vi "Producer Comsumer pattern.vi"() -> ()   [LabVIEW 2024]
panel:
  in  "stop":bool
  in  "Enqueue":bool
  out "Tank":dbl(slide) scale=0.0..10.0
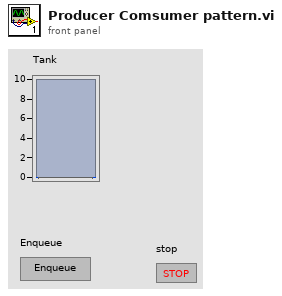
[diagram p1: front panel]
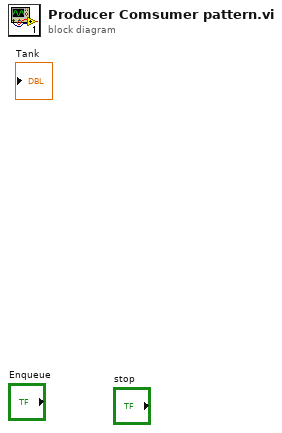
[diagram p0: block diagram]
diagram:
